vi "Test External Clock.vi"() -> ()   [LabVIEW 2021]
uses:
  Typedef/Clock History Map.ctl
  Typedef/Clock History.ctl
  Typedef/Timestamp Pair.ctl
  Typedef/Clock Conversion Map.ctl
  <vilib>/Platform/TimedLoop/XDataNode/timing_clust.ctl
  <vilib>/Platform/TimedLoop/XDataNode/nitl_modes.ctl
  <vilib>/Platform/TimedLoop/XDataNode/wakeup.ctl
  <vilib>/numeric/Random Number (Range) I64.vi
  Time Conversion/LabVIEW Time to UTC Time.vi
  CIFCore/Common/Utilities/Add Error.vi
  <vilib>/numeric/sub_Random U32.vi
  CIFCore/Common/Utilities/Append Error Location.vi
  <vilib>/platform/TimedLoop/XDataNode/XDataNode.xnode
  <vilib>/Platform/TimedLoop/XDataNode/XDNodeRunTimeDep.lvlib
  CIFClocks.lvlib
panel:
  out "error out":errorcluster
  out "Conversion error":i64
  out "Error (ns)":i64
  out "Waveform Chart 2":i64(graph)
  in  "stop":bool
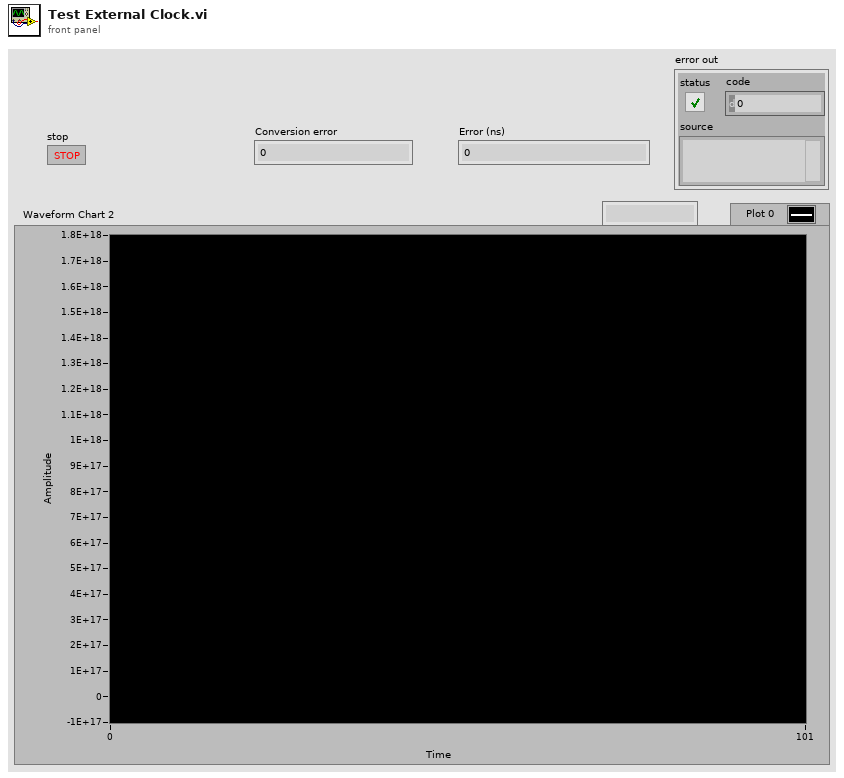
[diagram p1: front panel]
types:
  T1 = typedef "CIFClocks.lvlib/Clock Conversion Map.ctl" = map{u8, cluster{"Last Reset":u64, "Offset Pair":T2, "Slope":dbl}}
  T2 = typedef "CIFClocks.lvlib/Timestamp Pair.ctl" = cluster{"System Time":i64, "External Time":i64}
  T3 = typedef "CIFClocks.lvlib/Clock History Map.ctl" = map{u8, T4}
  T4 = typedef "CIFClocks.lvlib/Clock History.ctl" = cluster{"System Clock":i64[], "External Clock":i64[], "Last Reset Time":u64, "Slope":dbl[], "slope":dbl, "Offset Pair":T2}
  T5 = typedef "XDNodeRunTimeDep.lvlib/timing_clust.ctl" = cluster{"Expected End [f-1]":u64, "Actual End [f-1]":u64, "Finished Late? [f-1]":bool, "Expected End [i-1]":u64, "Actual End [i-1]":u64, "Finished Late? [i-1]":bool, "Expected Start [i]":u64, "Actual Start [i]":u64, "Expected Start [f]":u64, "Actual Start [f]":u64, "Source Name":string, "Structure Name":string, "Period":i64, "Deadline":i64, "Offset":i64, "Start":i64, "Priority":i32, "Timeout":i32, "Mode":T6, "Wakeup Reason":T7, "Error":errorcluster, "Source Type":string, "Secondary Source Type":string, "Global End Time":u64, "Global Start Time":u64, "Frame Duration":u64, "Iteration Duration":u64, "Assigned CPU":i32, "I/O Scan Engine Mode":u32}
  T6 = typedef "XDNodeRunTimeDep.lvlib/nitl_modes.ctl" = enum32{"No Change", "Process missed periods, maintain original phase", "Discard missed periods, maintain original phase", "Process missed periods, ignore original phase", "Discard missed periods, ignore original phase"}
  T7 = typedef "XDNodeRunTimeDep.lvlib/wakeup.ctl" = enum32{"Normal", "Aborted", "Asynchronous wakeup", "Timing source error", "Timed loop error", "Timeout"}
  T8 = typedef "CIFClocks.lvlib/Clock Conversion.ctl" = cluster{"ClockID":u8, "Last Reset":u64, "Offset Pair":T2, "Slope":dbl}
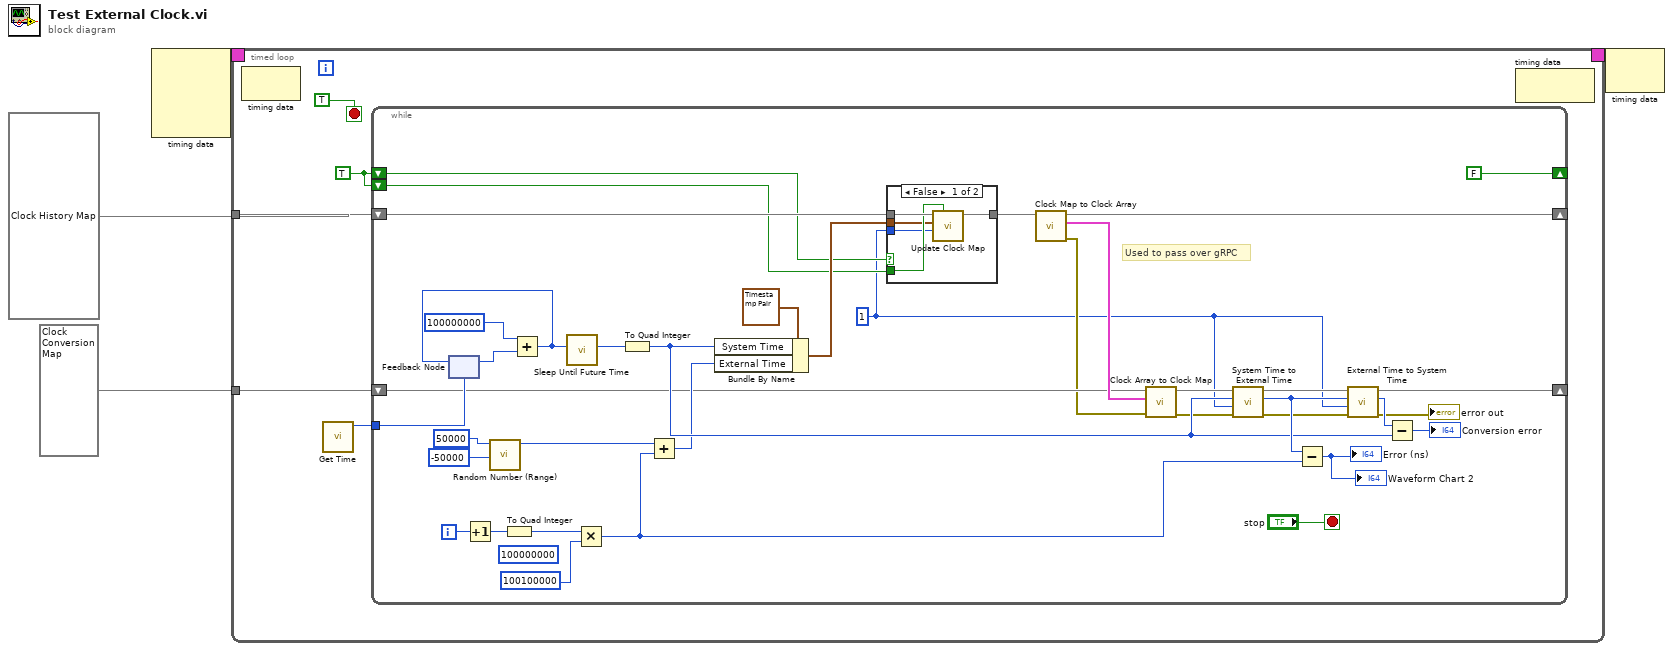
[diagram p0: block diagram]
diagram:
  n1 = node-c288() -> (w4:T5)  [unwired: 4 in]
  n2 = timed-loop {
    timing: w4 -> [_]
    timing-out: [_] -> w3
    tunnel: T3 {} ("Clock History Map in") -> [w7]
    tunnel: T1 {} ("Clock Convert Map out") -> [w5]
    stop <- TRUE stop-if-true
    w6 = TRUE
    n3 = node-c288() -> ()  [unwired: 1 in, 1 out]
    n4 = call "Get Time.vi"() -> ("Time (ns)"=w8:u64)  [unwired: 9 in, 2 out]
    n5 = while {
      tunnel: w8 -> [w45]
      shift-right: [w20] -> _
      shift-left: w7 -> [w40]
      shift-right: [FALSE] -> _
      shift-left: w6 -> [w35]
      shift-left: w6 -> [w34]
      shift-right: [w17] -> _
      shift-left: w5 -> [w16]
      i -> [w43]
      stop <- "stop" stop-if-true
      w10 = u8 1 ("ClockID")
      (unwired) i64 100000000 ("y")
      # "Used to pass over gRPC"
      n6 = feedback #1(w45) -> (w44:u64)
      n7 = Increment(x=w43) -> (x+1=w26:i32)
      n8 = call-poly <vilib>:"Random Number (Range).vi"("lower bound (-100)"=i64 -50000, "upper bound (100)"=i64 50000) -> ("number"=w15:i64)  [unwired: 9 in]
      n9 = To Quad Integer(1:w26) -> (0:w47:i64)
      n10 = Add(x=i64 100000000 ("y"), y=w44) -> (x+y=w37:u64)
      n11 = feedback-in #1(w37) -> ()
      n12 = call "Sleep Until Future Time.vi"("Wake Time"=w37) -> ("Wake Time (ns)"=w22:u64)  [unwired: 9 in, 1 out]
      n13 = Multiply(x=w47, y=i64 100100000) -> (x*y=w24:i64)
      n14 = To Quad Integer(1:w22) -> (0:w30:i64)
      n15 = Add(x=w15, y=w24) -> (x+y=w23:i64)
      n16 = Bundle By Name(cluster=T2 {"System Time"=1726494902617542000, "External Time"=44044000000} ("Timestamp Pair"), "System Time"=w30, "External Time"=w23) -> (w38:T2)
      n17 = case shown="False" w35 {
        tunnel: w40 -> [w52 w53]
        tunnel: w38 -> [w49 _]
        tunnel: [w51 w53] -> w21
        tunnel: w10 -> [w48 _]
        tunnel: w34 -> [w50 _]
        frame False {
          n18 = call "Update Clock Map.vi"("Reset"=w50, "ClockID"=w48, "Timestamp Pair"=w49, "Clock History Map in"=w52) -> ("Clock History Map out"=w51:map{u8, T4})  [unwired: 7 in]
        }
        frame True {
        }
      }
      n19 = call "Clock Map to Clock Array.vi"("Clock History Map in"=w21) -> ("error out"=w14:errorcluster, "Clock Conversion Array"=w19:T8[], "Clock History Map out"=w20:T3)  [unwired: 8 in]
      n20 = call "Clock Array to Clock Map.vi"("error in (no error)"=w14, "Clock Conversion Array"=w19, "Clock Convert Map in"=w16) -> ("error out"=w13:errorcluster, "Clock Convert Map out"=w18:T1)  [unwired: 7 in]
      n21 = call "System Time to External Time.vi"("error in (no error)"=w13, "ClockID"=w10, "System Time"=w30, "Clock Convert Map in"=w18) -> ("error out"=w12:errorcluster, "External Time"=w32:i64, "Clock Convert Map out"=w33:T1)  [unwired: 4 in, 1 out]
      n22 = Subtract(x=w32, y=w24) -> (x-y=→"Error (ns)" →"Waveform Chart 2":i64)
      n23 = call "External Time to System Time.vi"("error in (no error)"=w12, "ClockID"=w10, "External Time"=w32, "Clock Convert Map in"=w33) -> ("error out"=→"error out":errorcluster, "System Time"=w31:i64, "Clock Convert Map out"=w17:T1)  [unwired: 4 in, 1 out]
      n24 = Subtract(x=w31, y=w30) -> (x-y=→"Conversion error":i64)
    }
    n25 = node-c288() -> ()  [unwired: 1 in, 1 out]
  }
  n26 = node-c288(w3) -> ()  [unwired: 1 out]
